vi "AddAttribute.vi"(6 "Value":string, 8 "error in":errorcluster, 9 "Name":string, 10 "OwningElement in":refnum<k20>, 11 "Document in":refnum<k20>) -> (0 "error out":errorcluster, 2 "OwningElement out":refnum<k20>, 3 "Document out":refnum<k20>)   [LabVIEW 2021, in "ProligentXMLGenerator.lvlib" / "DOMSupport.lvlib"]
uses:
  DOMSupport.lvlib
  <resource>/objmgr/DOMUserDefRef.rc
  <vilib>/xml/NI_XML.lvlib
  <vilib>/xml/Close Reference(Node).vi
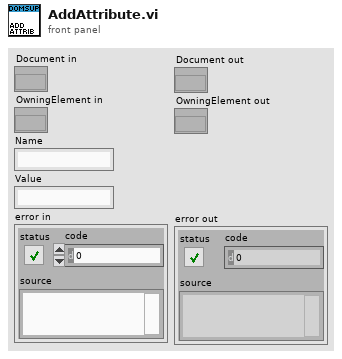
[diagram p1: front panel]
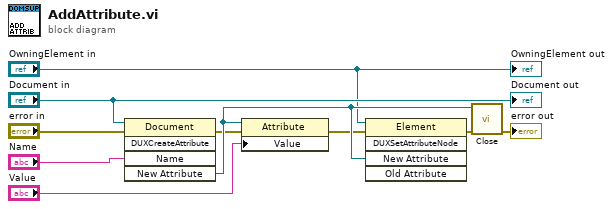
[diagram p0: block diagram]
diagram:
  n1 = invoke on="Invoke Node" class="Document" method="DUXCreateAttribute"(reference="Document in", error in="error in", "Name"="Name") -> (error out=w6:errorcluster, "New Attribute"=w10:refnum<k20>)  [unwired: 2 in, 3 out]
  n2 = property on="Property Node" class="Attribute "(reference=w10, error in=w6, "Value"="Value") -> (error out=w8:errorcluster)  [unwired: 1 out]
  n3 = invoke on="Invoke Node" class="Element" method="DUXSetAttributeNode"(reference="OwningElement in", error in=w8, "New Attribute"=w10) -> (error out=w7:errorcluster)  [unwired: 2 in, 4 out]
  n4 = call-poly <vilib>:"Close.vi"("error in (no error)"=w7, "node"=w10) -> ("error out"=→"error out":errorcluster)  [unwired: 7 in]
  "Document out" <- "Document in"
  "OwningElement out" <- "OwningElement in"
